vi "读取固件状态.vi"(8 "错误输入":errorcluster, 11 "MB session in":refnum<class "MB_Master.lvclass">) -> (0 "error out":errorcluster, 1 "固件状态":enum16{"正常", "砖头"}(ring), 2 "结果字符串":string, 3 "MB session out":refnum<class "MB_Master.lvclass">)   [LabVIEW 2022 SP3, in "斯坦道总氮.lvlib"]
uses:
  <vilib>/Plasmionique/MB Master/MB_Master/MB_Master.lvclass
  <vilib>/Plasmionique/MB Master/MB_Master_Serial/MB_Master_Serial.lvclass
  C:/Program Files (x86)/National Instruments/LabVIEW 2022/vi.lib/Plasmionique/MB Master/MB_Master/MB_Master.lvclass
  <vilib>/Plasmionique/MB Master/MB Master.lvlib
panel:
  in  "VISA Resource":refnum<visa-resource-name>
  in  "引用选择":enum16{"MB引用", "自建引用"}(ring)
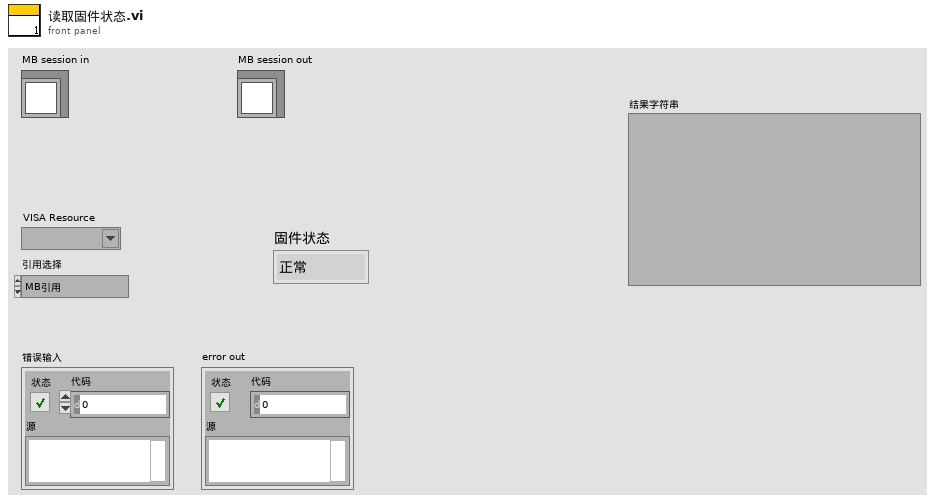
[diagram p1: front panel]
types:
  T1 = cluster{"baud rate (bps)":u32, "stop bits":u16, "parity":u16, "flow control":u16, "timeout":u32, "retries":i32}
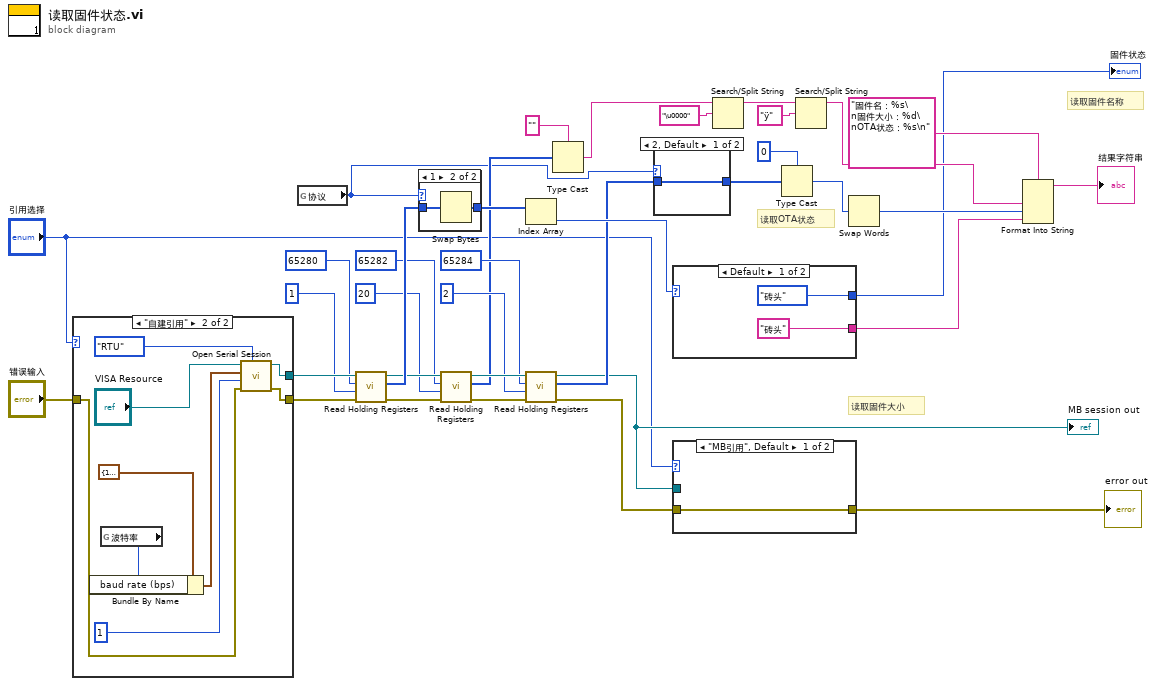
[diagram p0: block diagram]
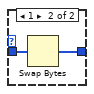
[diagram p2: hidden frame]
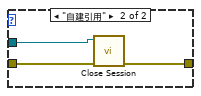
[diagram p4: hidden frame]
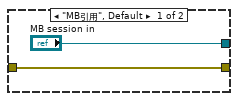
[diagram p5: hidden frame]
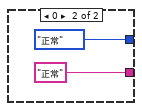
[diagram p6: hidden frame]
diagram:
  # "读取固件大小"
  # "读取固件名称"
  # "读取OTA状态"
  n1 = case shown="\"自建引用\"" "引用选择" {
    tunnel: ["MB session in" w47] -> w36
    tunnel: "错误输入" -> [w38 w46]
    tunnel: [w38 w45] -> w15
    frame "MB引用", Default {
    }
    frame "自建引用" {
      n2 = global read "总磷总氮断电保存全局变量.vi" "波特率"() -> (w42:u32)
      n3 = Bundle By Name(cluster=T1 {"baud rate (bps)"=115200, "stop bits"=10, "parity"=0, "flow control"=0, "timeout"=1000, "retries"=1} ("Serial Config"), "baud rate (bps)"=w42) -> (w40:T1)
      n4 = call <vilib>:"Open Serial Session.vi"("Mode (RTU)"=enum16{"RTU", "ASCII"}."RTU", "Error in"=w46, "Slave ID"=u8 1, "Serial Config"=w40, "VISA Resource"="VISA Resource") -> ("Error out"=w45:errorcluster, "MB_Serial session"=w47:refnum<class "MB_Master_Serial.lvclass">)  [unwired: 5 in]
    }
  }
  n5 = global read "总磷总氮断电保存全局变量.vi" "协议"() -> (w1:u16)
  n6 = call <vilib>:"Read Holding Registers.vi"("error in (no error)"=w15, "quantity"=u16 1, "starting address"=u16 65280, "MB session in"=w36) -> ("error out"=w23:errorcluster, "Registers"=w33:u16[], "MB session out"=w28:refnum<class "MB_Master.lvclass">)  [unwired: 5 in]
  n7 = case shown="1" w1 {
    tunnel: w33 -> [w49 w51]
    tunnel: [w49 w50] -> w31
    frame 2, Default {
    }
    frame 1 {
      n8 = Swap Bytes(anything=w51) -> (byte swapped=w50:u16[])
    }
  }
  n9 = call <vilib>:"Read Holding Registers.vi"("error in (no error)"=w23, "quantity"=u16 20, "starting address"=u16 65282, "MB session in"=w28) -> ("error out"=w22:errorcluster, "Registers"=w10:u16[], "MB session out"=w26:refnum<class "MB_Master.lvclass">)  [unwired: 5 in]
  n10 = Index Array(array=w31) -> (element=w32:u16)  [unwired: 1 in]
  n11 = call <vilib>:"Read Holding Registers.vi"("error in (no error)"=w22, "quantity"=u16 2, "starting address"=u16 65284, "MB session in"=w26) -> ("error out"=w8:errorcluster, "Registers"=w21:u16[], "MB session out"=w9:refnum<class "MB_Master.lvclass">)  [unwired: 5 in]
  "MB session out" <- w9
  n12 = Type Cast(type="", x=w10) -> (*(type *) &x=w11:string)
  n13 = case shown="2, Default" w1 {
    tunnel: w21 -> [w52 w54]
    tunnel: [w52 w53] -> w20
    frame 2, Default {
    }
    frame 1 {
      n14 = Swap Bytes(anything=w54) -> (byte swapped=w53:u16[])
    }
  }
  n15 = case shown="Default" w32 {
    tunnel: ["砖头" "正常"] -> w30
    tunnel: [enum16{"正常", "砖头"}."砖头" ("固件状态") enum16{"正常", "砖头"}."正常" ("固件状态")] -> w2
    frame Default {
    }
    frame 0 {
    }
  }
  "固件状态" <- w2
  n16 = case shown="\"MB引用\", Default" "引用选择" {
    tunnel: w9 -> [_ w62]
    tunnel: w8 -> [w59 w61]
    tunnel: [w59 w60] -> w7
    frame "MB引用", Default {
    }
    frame "自建引用" {
      n17 = call-dynamic "Close Session.vi"("error in (no error)"=w61, "MB session in"=w62) -> ("error out"=w60:errorcluster)  [unwired: 9 in]
    }
  }
  "error out" <- w7
  n18 = Search/Split String(string=w11, search string/char (-)="\u0000" ("搜索字符串")) -> (substring before match=w5:string)  [unwired: 1 in, 2 out]
  n19 = Type Cast(type=u32 0, x=w20) -> (*(type *) &x=w18:u32)
  n20 = Search/Split String(string=w5, search string/char (-)="ÿ" ("搜索字符串")) -> (substring before match=w4:string)  [unwired: 1 in, 2 out]
  n21 = Swap Words(1:w18) -> (0:w17:u32)
  n22 = Format Into String(format string="固件名：%s\n固件大小：%d\nOTA状态：%s\n" ("格式字符串"), w4, w17, w30) -> (resulting string=→"结果字符串":string)  [unwired: 2 in, 1 out]
